vi "deinitialize.vi"(0 "HGF_Queue":refnum<class "HGF_Queue.lvclass">, 5 "error in (no error)":errorcluster) -> (19 "error out":errorcluster)   [LabVIEW 2014, in "HGF_BaseClasses.lvlib" / "HGF_Queue.lvclass"]
doc: "This is a dynamic dispatch VI. It can be overwritten by childclasses to release allocated recources."
uses:
  HGF_Queue.lvclass
  HGF_TriggeredEvent/HGF_TriggeredEvent.lvclass
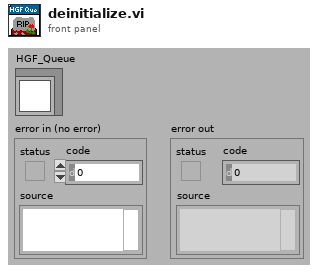
[diagram p1: front panel]
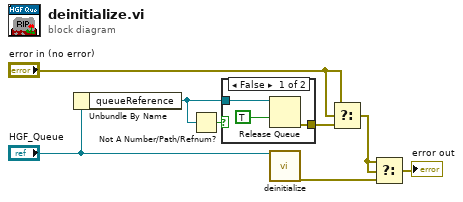
[diagram p0: block diagram]
diagram:
  n1 = Unbundle By Name("HGF_Queue") -> ("queueReference"=w1:refnum<queue>)
  n2 = Not A Number/Path/Refnum?(number/path/refnum=w1) -> (NaN/Path/Refnum?=w2:bool)
  n3 = case shown="False" w2 {
    tunnel: w1 -> [w11 _]
    tunnel: [w9 _] -> w6
    frame False {
      n4 = Release Queue(queue=w11, force destroy? (F)=TRUE) -> (error out=w9:errorcluster)  [unwired: 1 in, 2 out]
    }
    frame True {
    }
  }
  n5 = call-parent "deinitialize.vi"("HGF_Factory"="HGF_Queue") -> ("error out"=w5:errorcluster)  [unwired: 1 in, 17 out]
  n6 = Select(t="error in (no error)", s="error in (no error)", f=w6) -> (s? t:f=w4:errorcluster)
  n7 = Select(t=w4, s=w4, f=w5) -> (s? t:f=→"error out":errorcluster)
